vi "is a.vi"(8 "error in (no error)":errorcluster, 11 "Hardware in":refnum<class "Hardware.lvclass">) -> (0 "error out":errorcluster, 2 "is a":string, 3 "Hardware out":refnum<class "Hardware.lvclass">)   [LabVIEW 2016, in "Hardware.lvlib" / "Hardware.lvclass"]
uses:
  <userlib>/Common Components/Hardware/Abstract Hardware/Hardware.lvclass
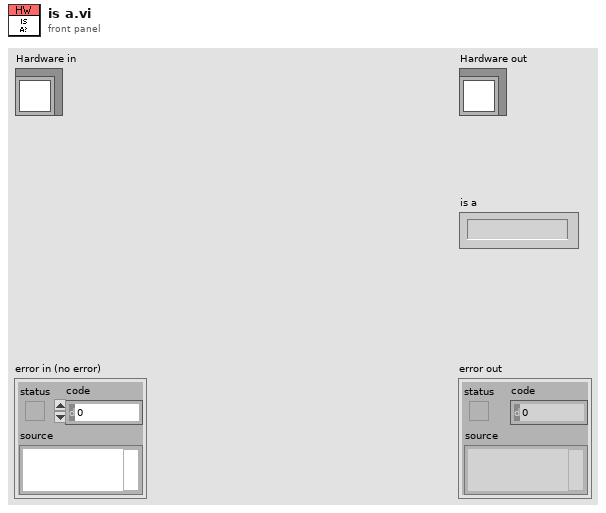
[diagram p1: front panel]
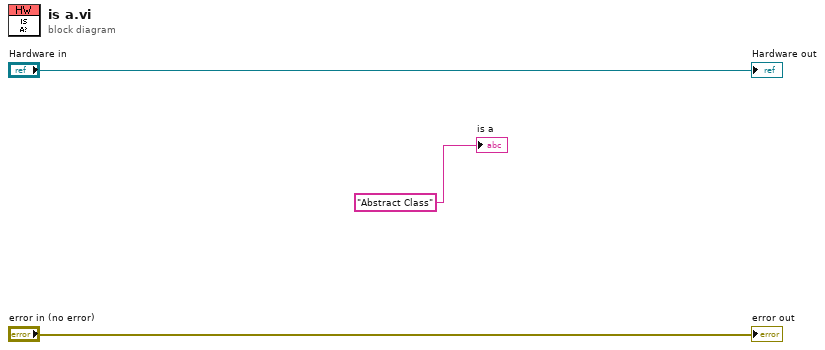
[diagram p0: block diagram]
diagram:
  "error out" <- "error in (no error)"
  "Hardware out" <- "Hardware in"
  "is a" <- "Abstract Class" ("is a")
